vi "Draw.vi"(8 "error in (no error)":errorcluster, 11 "TileTimer in":refnum<class "TileTimer.lvclass">) -> (0 "error out":errorcluster, 3 "TileTimer out":refnum<class "TileTimer.lvclass">)   [LabVIEW 2019, in "RT_Game.lvlib" / "TileTimer.lvclass"]
uses:
  TileTimer.lvclass
  C:/Users/FreshBob/Dropbox/VIs/myRIO_GameConsole/RT/RT_Game/GameObject/GameObject.lvclass
  Color.ctl
  GameObject/GameObject.lvclass/GameObject.ctl
  TileTimer.lvclass/TileTimer.ctl
  GameObject/Read position.vi
  Engine/Engine.lvclass
  RT_Game.lvlib
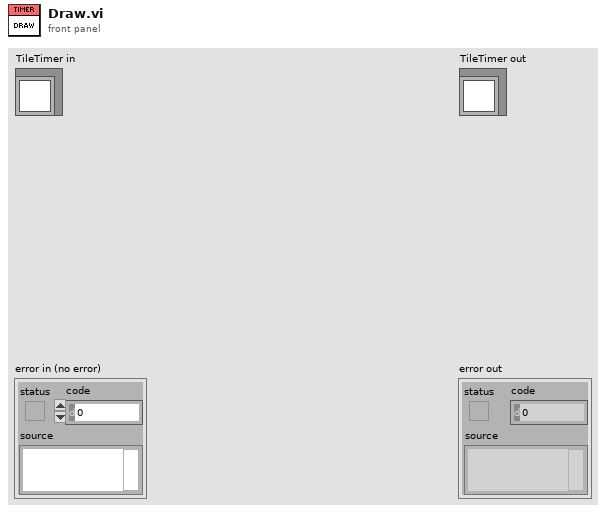
[diagram p1: front panel]
types:
  T1 = typedef "RT_Game.lvlib/Color.ctl" = fxp<+,3,3>
  T2 = typedef "RT_Game.lvlib/Game.lvclass/Coordinate.ctl" = cluster{"x":dbl, "y":dbl}
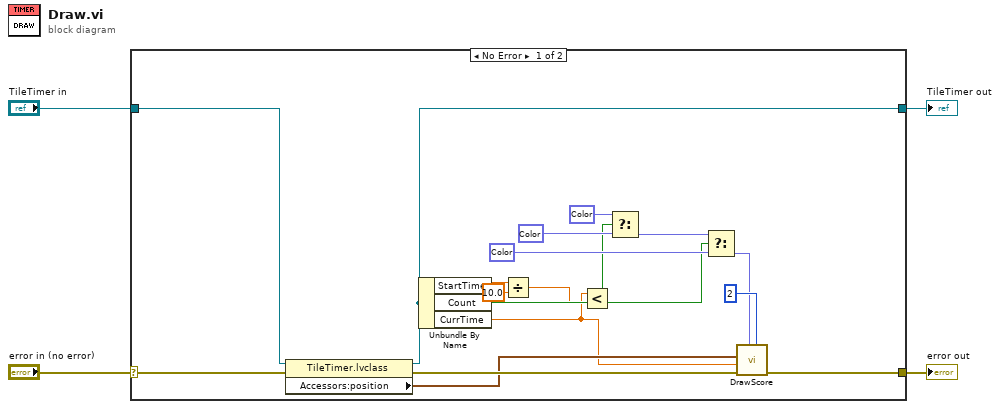
[diagram p0: block diagram]
diagram:
  n1 = case shown="No Error" "error in (no error)" {
    selector: "error in (no error)" -> [w22 w24]
    tunnel: [w21 w24] -> w3
    tunnel: [w15 w23] -> w1
    tunnel: "TileTimer in" -> [w19 w23]
    frame No Error {
      n2 = property class="TileTimer.lvclass"(reference=w19, error in=w22) -> (reference out=w15:refnum<class "TileTimer.lvclass">, error out=w20:errorcluster, "Accessors:position"=w18:T2)
      n3 = Unbundle By Name(w15) -> ("StartTime"=w10:dbl, "Count"=w13:bool, "CurrTime"=w11:dbl)
      n4 = Divide(x=w10, y=10.0) -> (x/y=w8:dbl)
      n5 = Less?(x=w11, y=w8) -> (x < y?=w6:bool)
      n6 = Select(t=T1 1.0, s=w6, f=T1 2.0 ("t")) -> (s? t:f=w7:T1)
      n7 = Select(t=w7, s=w13, f=T1 7.0 ("Color")) -> (s? t:f=w14:T1)
      n8 = call "DrawScore.vi"("Digits"=2, "Color"=w14, "error in (no error)"=w20, "score"=w11, "position"=w18) -> ("error out"=w21:errorcluster)  [unwired: 6 in]
    }
    frame Error {
    }
  }
  "error out" <- w3
  "TileTimer out" <- w1
